vi "SetExternalInterfaces.vi"(8 "Error In":errorcluster, 10 "ExternalInterfaces":T1[](array[typedef]), 11 "reference in":refnum<class "TraceWindow.lvclass">) -> (0 "Error Out":errorcluster, 3 "reference out":refnum<class "TraceWindow.lvclass">)   [LabVIEW 2021, in "TraceWindow.lvlib" / "TraceWindow.lvclass"]
uses:
  TraceWindow.lvclass
  Library_TAF_Support/ClusterArrayConversion/BundledArray.ctl
  0a6ec689-4898-488c-8e07-ed5616c8d135.vi
  Library_TAF_Support/ClusterArrayConversion/ClusterArrayConversion.lvlib
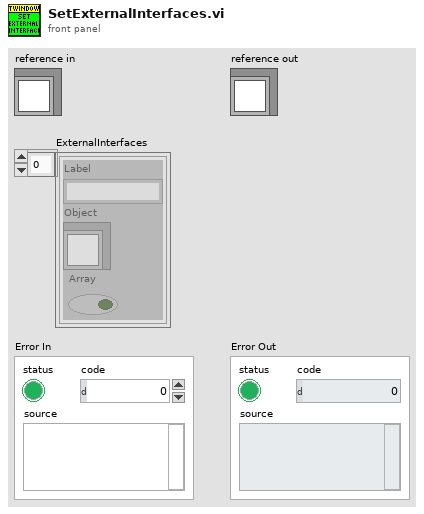
[diagram p1: front panel]
types:
  T1 = typedef "ClusterArrayConversion.lvlib/BundledArray.ctl" = cluster{"Label":string, "Object":refnum<class>, "Array":bool}
  T2 = typedef "TraceWindow.lvlib/TraceWindow.lvclass/ObjectAttributes.ctl" = cluster{"Interfaces":cluster{"Dummys":refnum<class>}, "Locals":cluster{"MainGUIActive":refnum<queue>, "TraceQueue":refnum<queue>}, "Persistent":cluster{"OpenAtClosure":bool, "BufferSize":i32, "Startup":cluster{"OpenAtStartUp":bool, "OpenMinimized":bool}}}
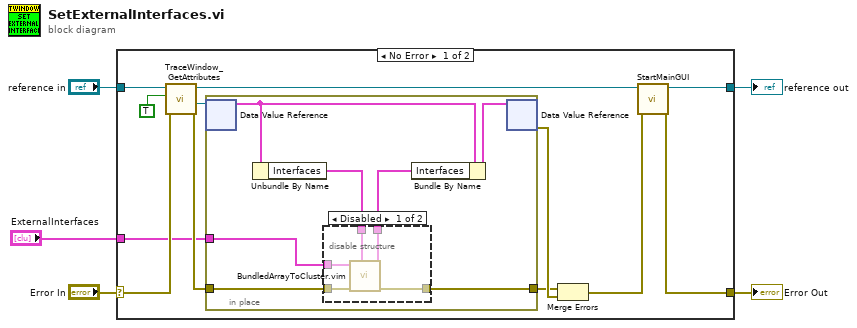
[diagram p0: block diagram]
diagram:
  n1 = case shown="No Error" "Error In" {
    selector: "Error In" -> [w15 w31]
    tunnel: [w6 w31] -> w4
    tunnel: [w8 w30] -> w2
    tunnel: "reference in" -> [w17 w30]
    tunnel: "ExternalInterfaces" -> [w9 _]
    frame No Error {
      n2 = call "TraceWindow_GetAttributes.vi"("error in (no error)"=w15, "OnlyGetDvrReference(False)"=TRUE, "reference in"=w17) -> ("error out"=w10:errorcluster, "DataRef"=w12:refnum<data-value>, "reference out"=w16:refnum<class "TraceWindow.lvclass">)  [unwired: 5 in, 1 out]
      n3 = in-place {
        in-place-border: [w23] -> w11
        in-place-border: w10 -> [w18]
        in-place-border: w9 -> [w19]
        n4 = in-place-dvr #1(w12) -> (w22:T2)  [unwired: 1 out]
        n5 = Unbundle By Name(w22) -> ("Interfaces"=w21:cluster{"Dummys":refnum<class>})
        n6 = disable-structure shown="Disabled" {
          disable-tunnel: [w29 _] -> w23
          disable-tunnel: w21 -> [w28 _]
          disable-tunnel: [w27 _] -> w20
          disable-tunnel: w19 -> [w26 _]
          disable-tunnel: w18 -> [w25 _]
          frame Disabled {
            n7 = call "BundledArrayToCluster.vim"("Type"=w28, "error in (no error)"=w25, "BundeledLabels"=w26) -> ("error out"=w29:errorcluster, "DataOut"=w27:cluster{"Dummys":refnum<class>})  [unwired: 7 in]
          }
          frame Enabled {
          }
        }
        n8 = Bundle By Name(cluster=w22, "Interfaces"=w20) -> (w24:T2)
        n9 = in-place-dvr #1(w24) -> (w13:errorcluster)  [unwired: 1 out]
      }
      n10 = Merge Errors(w11, w13) -> (w7:errorcluster)
      n11 = call "StartMainGUI.vi"("Error In"=w7, "reference in"=w16) -> ("Error Out"=w6:errorcluster, "reference out"=w8:refnum<class "TraceWindow.lvclass">)  [unwired: 6 in, 2 out]
    }
    frame Error {
    }
  }
  "Error Out" <- w4
  "reference out" <- w2
